vi "Calculate_2.vi"(11 "Operators":string[](array[string])) -> (2 "Value Out":u64, 3 "Operators Out":string[](array[string]))   [LabVIEW 2018]
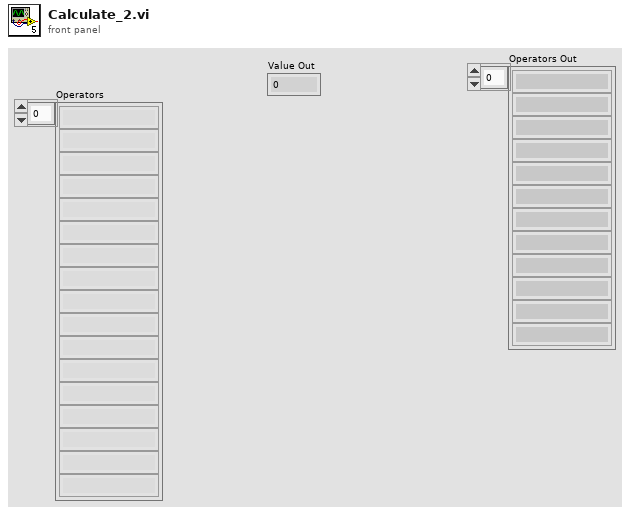
[diagram p1: front panel]
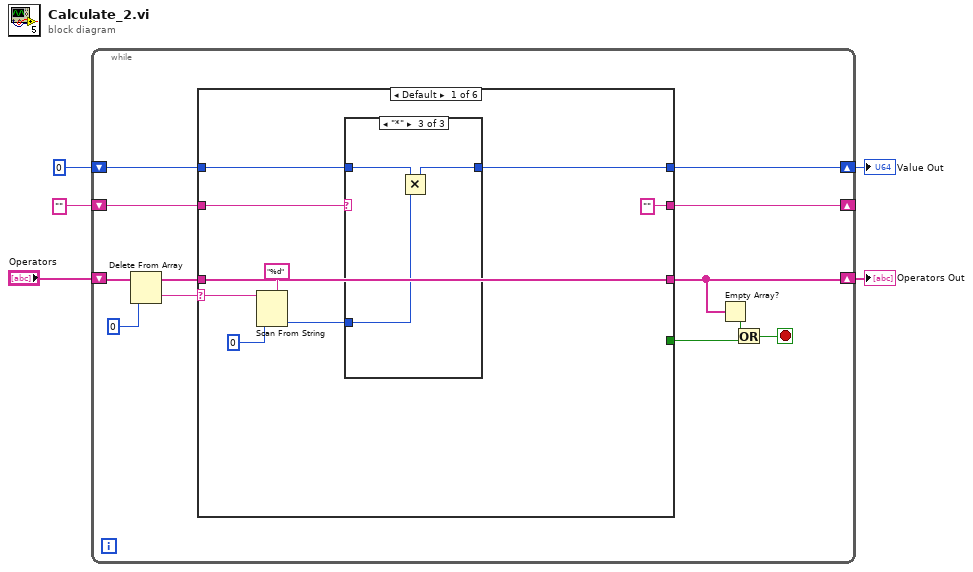
[diagram p0: block diagram]
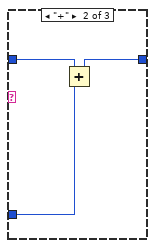
[diagram p3: hidden frame]
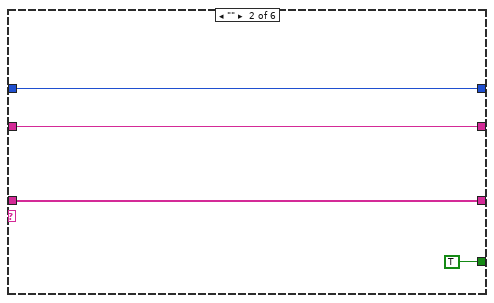
[diagram p4: hidden frame]
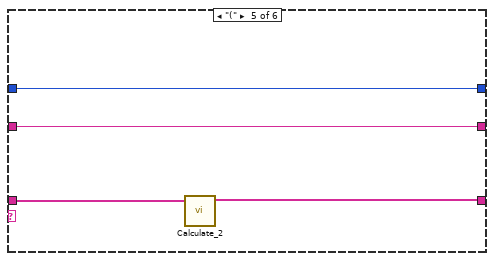
[diagram p7: hidden frame]
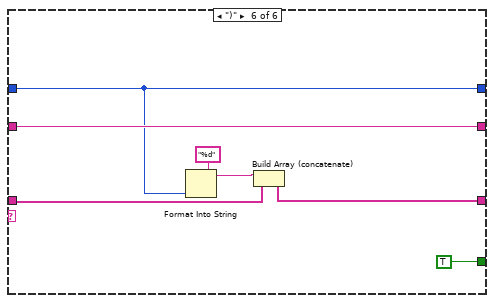
[diagram p8: hidden frame]
diagram:
  n1 = while {
    shift-right: [w6] -> w2
    shift-left: u64 0 -> [w15]
    shift-right: [w17] -> _
    shift-left: "" -> [w16]
    shift-right: [w10] -> w1
    shift-left: "Operators" -> [w14]
    stop <- w8 stop-if-true
    n2 = Delete From Array(array=w14, index=0) -> (deleted portion=w12:string, array with subset deleted=w11:string[])  [unwired: 1 in]
    n3 = case shown="Default" w12 {
      selector: w12 -> [w23 _ w39 w43 _ _]
      tunnel: ["" w35 w39 w43 w44 w54] -> w17
      tunnel: w16 -> [w26 w35 _ _ w44 w54]
      tunnel: [w20 w34 w40 w42 w45 w53] -> w6
      tunnel: w15 -> [w25 w34 w40 w42 w45 w53]
      tunnel: w11 -> [w18 w36 w38 w41 w47 w50]
      tunnel: [w18 w36 w38 w41 w46 w49] -> w10
      tunnel: [_ TRUE _ _ _ TRUE] -> w7
      frame Default {
        n4 = Scan From String(format string="%d", input string=w23, default 1=u64 0) -> (output 1=w21:u64)  [unwired: 2 in, 3 out]
        n5 = case shown="\"*\"" w26 {
          tunnel: w25 -> [_ w30 w33]
          tunnel: w21 -> [w27 w29 w32]
          tunnel: [w27 w28 w31] -> w20
          frame Default {
          }
          frame "+" {
            n6 = Add(x=w30, y=w29) -> (x+y=w28:u64)
          }
          frame "*" {
            n7 = Multiply(x=w33, y=w32) -> (x*y=w31:u64)
          }
        }
      }
      frame "" {
      }
      frame "+" {
      }
      frame "*" {
      }
      frame "(" {
        n8 = call "Calculate_2.vi"("Operators"=w47) -> ("Operators Out"=w46:string[])  [unwired: 9 in, 1 out]
      }
      frame ")" {
        n9 = Format Into String(format string="%d", w53) -> (resulting string=w51:string)  [unwired: 2 in, 1 out]
        n10 = Build Array (concatenate)(w51, w50) -> (w49:string[])
      }
    }
    n11 = Empty Array?(array=w10) -> (empty?=w9:bool)
    n12 = Or(x=w9, y=w7) -> (x .or. y?=w8:bool)
  }
  "Value Out" <- w2
  "Operators Out" <- w1
